vi "Movement test.vi"() -> ()   [LabVIEW 2018]
uses:
  Type Defs/The Motion Parameters.ctl
  Type Defs/G Code Command Cluster.ctl
  <vilib>/Motion/Express/_s/nimc.ex.resetPosition.resetPosition.axis.vi
  <vilib>/Motion/Express/_s/nimc.ex.straightLineMove.startStraightLineMove.coordinate.modeAbsolute.blendEnable.1.vi
  <vilib>/Motion/BlockNode/FB.NIMotion.xnode
  <vilib>/Motion/Express/_s/nimc.fb.straightLineMove.blendMode.ctl
panel:
  in  "resource":refnum<k21>
  out "error out":errorcluster
  in  "G0 Velocity":dbl=10.0
  in  "G Code":T1
  in  "Motion Parameters":T2={"Timeout"=1.0, "Blend Mode"=10551334, "Acceleration"=5.0, "Deceleration"=5.0, "Accel. Jerk"=2.0, "Decel. Jerk"=2.0, "Smoothing"=0.5, "Last Blend"=FALSE, "Blend Delay"=-1.0} {"Blend Delay" format="%#_13g"; "Decel. Jerk" format="%#_13g"; "Blend Mode" items=["At Profile Complete"=10551335, "At Deceleration"=10551334, "After Delay"=10551336]}
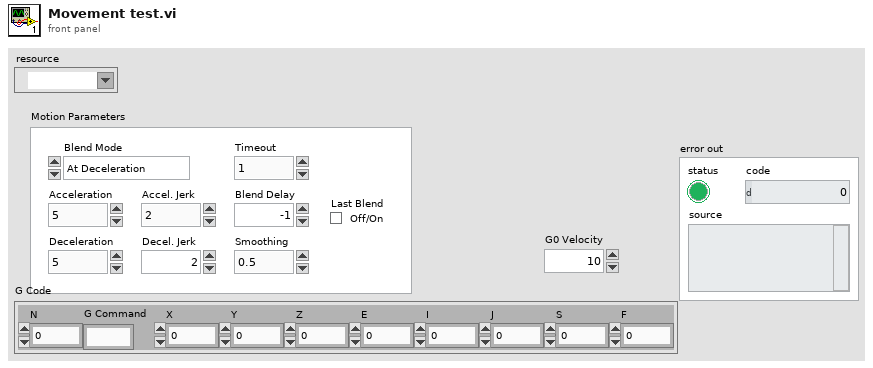
[diagram p1: front panel]
types:
  T1 = typedef "G Code Command Cluster.ctl" = cluster{"N":dbl, "G Command":string, "X":dbl, "Y":dbl, "Z":dbl, "E":dbl, "I":dbl, "J":dbl, "S":dbl, "F":dbl}
  T2 = typedef "The Motion Parameters.ctl" = cluster{"Timeout":dbl, "Blend Mode":i32, "Acceleration":dbl, "Deceleration":dbl, "Accel. Jerk":dbl, "Decel. Jerk":dbl, "Smoothing":dbl, "Last Blend":bool, "Blend Delay":dbl}
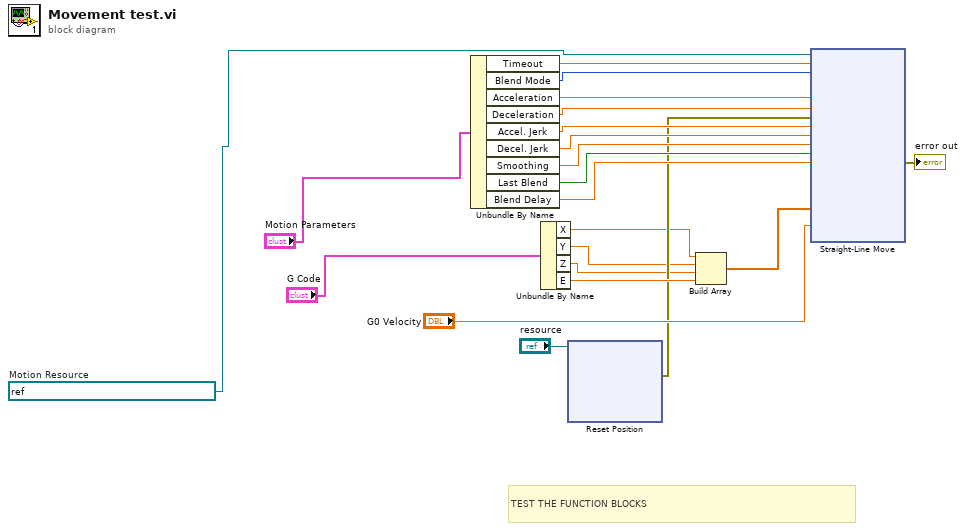
[diagram p0: block diagram]
diagram:
  w7 = refnum<k21> "nism://NI-cRIO9024/Printer Space"  # Motion Resource
  # "TEST THE FUNCTION BLOCKS"
  n1 = Unbundle By Name("Motion Parameters") -> ("Timeout"=w13:dbl, "Blend Mode"=w14:i32, "Acceleration"=w15:dbl, "Deceleration"=w16:dbl, "Accel. Jerk"=w17:dbl, "Decel. Jerk"=w18:dbl, "Smoothing"=w19:dbl, "Last Blend"=w20:bool, "Blend Delay"=w21:dbl)
  n2 = Unbundle By Name("G Code") -> ("X"=w1:dbl, "Y"=w2:dbl, "Z"=w3:dbl, "E"=w8:dbl)
  n3 = xnode ("Reset Position")("resource"="resource") -> ("error out"=w5:errorcluster)  [unwired: 2 in, 1 out]
  n4 = Build Array(w1, w2, w3, w8) -> (w12:dbl[])
  n5 = xnode ("Straight-Line Move")("position[]"=w12, "velocity"="G0 Velocity", "resource"=w7, "timeout"=w13, "blend mode"=w14, "acceleration"=w15, "deceleration"=w16, "error in"=w5, "accel. jerk"=w17, "decel. jerk"=w18, "smoothing"=w19, "last blend"=w20, "blend delay"=w21) -> ("error out"=→"error out":errorcluster)  [unwired: 2 out]
